vi "Add Virtual Instruments.vi"(8 "error in":errorcluster, 10 "<JSON CFG>":string, 11 "MSS in":refnum<class "Measure and Stimulus Subsystems.lvclass">) -> (0 "error out":errorcluster, 1 "Target Virt Instrs":T1(array[cluster]), 3 "MSS out":refnum<class "Measure and Stimulus Subsystems.lvclass">)   [LabVIEW 2023, in "HAL GOOP4.lvlib" / "Measure and Stimulus Subsystems.lvclass"]
uses:
  Measure and Stimulus Subsystems.lvclass
  0659c67a-1773-4fc6-81d6-9a69799a16e9.vi
  <vilib>/JDP Science/JSONtext/Find Item.vi
  <vilib>/JDP Science/JSONtext/Next JSON Value.vi
  <vilib>/JDP Science/JSONtext/String Subset.vi
  <vilib>/JDP Science/JSONtext/Parsing/Advance past next JSON Value (inlined COPY).vi
  <vilib>/JDP Science/JSONtext/Parsing/Advance past whitespace.vi
  <vilib>/JDP Science/JSONtext/Parsing/Advance past String.vi
  <vilib>/JDP Science/JSONtext/Parsing/Advance past Number.vi
  <vilib>/JDP Science/JSONtext/Parsing/Advance past Line Ending.vi
  <vilib>/JDP Science/JSONtext/Parsing/Parse Full Path or Item Name.vi
  <vilib>/JDP Science/JSONtext/Parsing/Advance past Array.vi
  <vilib>/JDP Science/JSONtext/Parsing/Advance past Object.vi
  <vilib>/JDP Science/JSONtext/support/Error Cluster From Code.vi
  <vilib>/JDP Science/JSONtext/Offset/Find Item Locations by Path.vi
  <vilib>/JDP Science/JSONtext/JSON text to Variant.vi
  <vilib>/Utility/error.llb/Error Cluster From Error Code.vi
  <vilib>/JDP Science/JSONtext/LVClass Serializer/JSONtext LVClass Serializer.lvclass
  <vilib>/ErrorRing/Error Ring.xnode
  Measure and Stimulus Subsystems.lvclass/Measure and Stimulus Subsystems.ctl
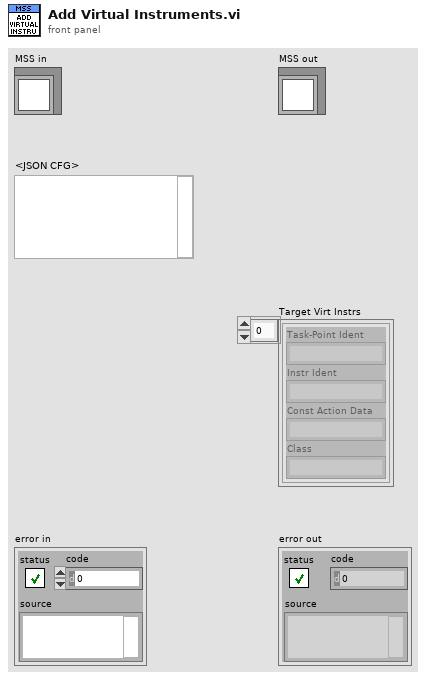
[diagram p1: front panel]
types:
  T1 = cluster{"Task-Point Ident":string, "Instr Ident":string, "Const Action Data":string, "Class":string}[]
  T2 = cluster{"Point Ident":string, "Instr Ident":string, "Const Action Data":string, "Class":string}[]
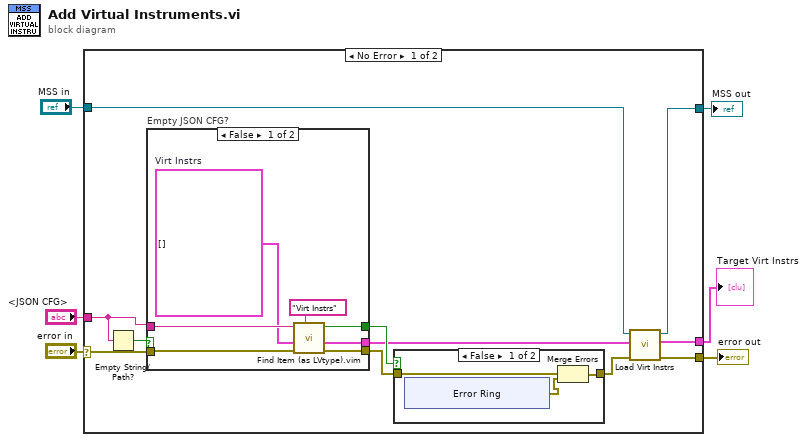
[diagram p0: block diagram]
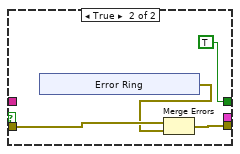
[diagram p3: hidden frame]
diagram:
  n1 = case shown="No Error" "error in" {
    selector: "error in" -> [w8 w44]
    tunnel: [w17 w43] -> w6
    tunnel: [w16 w44] -> w5
    tunnel: "MSS in" -> [w12 w43]
    tunnel: "<JSON CFG>" -> [w9 _]
    tunnel: [w7 _] -> w1
    frame No Error {
      n2 = Empty String/Path?(string/path=w9) -> (empty?=w15:bool)
      n3 = case "Empty JSON CFG?" shown="False" w15 {
        tunnel: w8 -> [w33 w37]
        tunnel: [w31 w35] -> w13
        tunnel: w9 -> [w32 _]
        tunnel: [w28 _] -> w10
        tunnel: [w27 TRUE ("Found")] -> w14
        frame False {
          w30 = T2 []  # Virt Instrs
          n4 = call "Find Item (as LVtype).vim"("$Path or Item Name"="Virt Instrs", "error in (no error)"=w33, "Data Type and Default Value"=w30, "JSON"=w32) -> ("error out"=w31:errorcluster, "Data"=w28:T2, "Found"=w27:bool)  [unwired: 4 in, 1 out]
        }
        frame True {
          n5 = xnode "Error Ring"() -> ("error out"=w36:errorcluster)
          n6 = Merge Errors(w37, w36) -> (w35:errorcluster)
        }
      }
      n7 = case shown="False" w14 {
        tunnel: [w20 w26] -> w11
        tunnel: w13 -> [w18 w26]
        frame False {
          n8 = xnode "Error Ring"() -> ("error out"=w19:errorcluster)
          n9 = Merge Errors(w18, w19) -> (w20:errorcluster)
        }
        frame True {
        }
      }
      n10 = call "Load Virt Instrs.vi"("error in"=w11, "Virt Instrs"=w10, "MSS in"=w12) -> ("error out"=w16:errorcluster, "Target Virt Instrs"=w7:T1, "MSS out"=w17:refnum<class "Measure and Stimulus Subsystems.lvclass">)  [unwired: 6 in]
    }
    frame Error {
    }
  }
  "error out" <- w5
  "MSS out" <- w6
  "Target Virt Instrs" <- w1
